vi "distance from ball to basket center.vi"(3 "d":dbl, 4 "alpha":dbl, 5 "theta":dbl) -> (0 "horizontal D2T [m]":dbl, 1 "Vertical D2T [m]":dbl, 2 "d2t":dbl)   [LabVIEW 2011]
uses:
  <vilib>/express/express arith-compare/Formula/XNode/ExpressFormulaBlockNode.xnode
panel:
  in  "is bottom?":bool=TRUE
  # "degrees"
  # "meters"
  # "all units are in meters and degrees"
  # "degrees"
  # "meters"
  # "t"
  # "d2t"
  # "p"
  # "w"
  # "d"
  # "fi"
  # "f"
  # "theta"
  # "h"
  # "beta"
  # "w - canon width\nh - canon height\ns - canon lowest point to camera viewing point - y\nt - distance from basket center to backboard center - y\np - distance from basket center to backboard center - x"
  # "s"
  # "alpha"
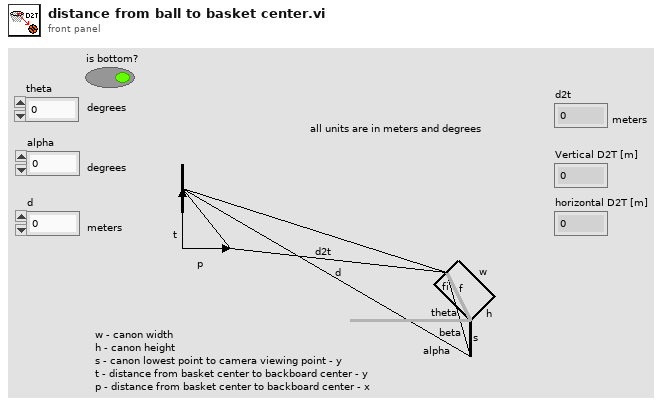
[diagram p1: front panel]
types:
  T1 = cluster{"canon height":dbl, "canon width":dbl, "distance from basket center to backboard center - x":dbl, "distance from basket center to backboard center - y":dbl, "canon lowest point to camera viewing point - y":dbl}
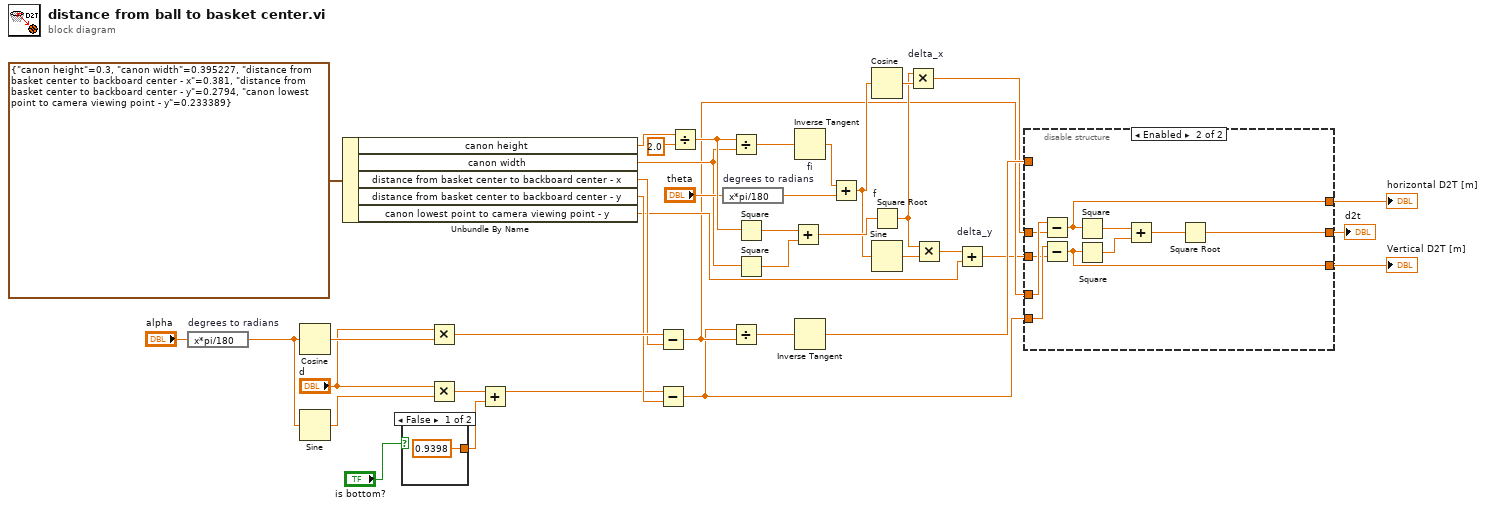
[diagram p0: block diagram]
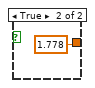
[diagram p2: hidden frame]
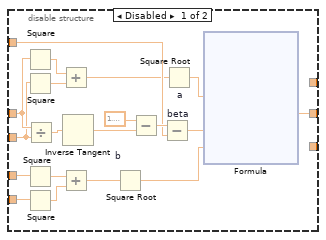
[diagram p3: hidden frame]
diagram:
  n1 = expression code="x*pi/180" "degrees to radians"("alpha") -> (w12:dbl)
  n2 = Cosine(x=w12) -> (cos(x)=w25:dbl)
  n3 = Sine(x=w12) -> (sin(x)=w23:dbl)
  n4 = Unbundle By Name(T1 {"canon height"=0.3, "canon width"=0.395227, "distance from basket center to backboard center - x"=0.381, "distance from basket center to backboard center - y"=0.2794, "canon lowest point to camera viewing point - y"=0.233389}) -> ("canon height"=w19:dbl, "canon width"=w18:dbl, "distance from basket center to backboard center - x"=w17:dbl, "distance from basket center to backboard center - y"=w16:dbl, "canon lowest point to camera viewing point - y"=w11:dbl)
  n5 = case shown="False" "is bottom?" {
    tunnel: [0.9398 ("y") 1.778 ("y")] -> w2
    frame False {
    }
    frame True {
    }
  }
  n6 = Multiply(x="d", y=w25) -> (x*y=w21:dbl)
  n7 = Multiply(x="d", y=w23) -> (x*y=w22:dbl)
  n8 = Add(x=w22, y=w2) -> (x+y=w3:dbl)
  n9 = Subtract(x=w21, y=w17) -> (x-y=w10:dbl)
  n10 = Subtract(x=w3, y=w16) -> (x-y=w8:dbl)
  n11 = Divide(x=w19, y=2.0) -> (x/y=w35:dbl)
  n12 = expression code="x*pi/180" "degrees to radians"("theta") -> (w31:dbl)
  n13 = Divide(x=w35, y=w18) -> (x/y=w34:dbl)
  n14 = Divide(x=w8, y=w10) -> (x/y=w15:dbl)
  n15 = Square(x=w35) -> (x^2=w38:dbl)
  n16 = Square(x=w18) -> (x^2=w37:dbl)
  n17 = Add(x=w38, y=w37) -> (x+y=w36:dbl)
  n18 = Inverse Tangent "fi"(1:w34) -> (0:w33:dbl)
  n19 = Inverse Tangent ("fi")(1:w15) -> (0:w14:dbl)
  n20 = Add(x=w33, y=w31) -> (x+y=w30:dbl)
  n21 = Cosine(x=w30) -> (cos(x)=w29:dbl)
  n22 = Square Root "f"(x=w36) -> (sqrt(x)=w28:dbl)
  n23 = Sine(x=w30) -> (sin(x)=w27:dbl)
  n24 = Multiply "delta_x"(x=w28, y=w29) -> (x*y=w9:dbl)
  n25 = Multiply(x=w28, y=w27) -> (x*y=w26:dbl)
  n26 = Add "delta_y"(x=w26, y=w11) -> (x+y=w7:dbl)
  n27 = disable-structure shown="Enabled" {
    disable-tunnel: w14 -> [w53 _]
    disable-tunnel: w10 -> [w46 w78]
    disable-tunnel: w9 -> [w45 w77]
    disable-tunnel: w8 -> [w44 w76]
    disable-tunnel: w7 -> [w43 w75]
    disable-tunnel: [w42 w79] -> w6
    disable-tunnel: [_ w74] -> w5
    disable-tunnel: [_ w73] -> w4
    frame Disabled {
      n28 = Square(x=w45) -> (x^2=w52:dbl)
      n29 = Square(x=w43) -> (x^2=w51:dbl)
      n30 = Square(x=w46) -> (x^2=w57:dbl)
      n31 = Square(x=w44) -> (x^2=w56:dbl)
      n32 = Divide(x=w45, y=w43) -> (x/y=w60:dbl)
      n33 = Add(x=w52, y=w51) -> (x+y=w50:dbl)
      n34 = Add(x=w57, y=w56) -> (x+y=w55:dbl)
      n35 = Inverse Tangent ("fi")(1:w60) -> (0:w58:dbl)
      n36 = Square Root "b"(x=w55) -> (sqrt(x)=w47:dbl)
      n37 = Subtract(x=1.5707963267948966, y=w58) -> (x-y=w54:dbl)
      n38 = Subtract "beta"(x=w54, y=w53) -> (x-y=w49:dbl)
      n39 = Square Root "a"(x=w50) -> (sqrt(x)=w48:dbl)
      n40 = xnode "Formula"("a"=w48, "beta"=w49, "b"=w47) -> ("Result"=w42:dbl)  [unwired: 1 in, 1 out]
    }
    frame Enabled {
      n41 = Subtract(x=w78, y=w77) -> (x-y=w74:dbl)
      n42 = Subtract(x=w76, y=w75) -> (x-y=w73:dbl)
      n43 = Square(x=w74) -> (x^2=w80:dbl)
      n44 = Square(x=w73) -> (x^2=w81:dbl)
      n45 = Add(x=w80, y=w81) -> (x+y=w82:dbl)
      n46 = Square Root(x=w82) -> (sqrt(x)=w79:dbl)
    }
  }
  "d2t" <- w6
  "horizontal D2T [m]" <- w5
  "Vertical D2T [m]" <- w4
